vi "LabVIEW host computer v1.0.vi"() -> ()   [LabVIEW 2015]
uses:
  <vilib>/Instr/_visa.llb/VISA Configure Serial Port (Instr).vi
panel:
  out "CH1/CH2":dbl
  out "ch2 dBm":dbl(graph)
  out "XW":string
  out "ch2 Power":dbl(graph)
  out "ch2 Power":dbl
  out "ch2 dB":dbl(graph)
  out "ch2 dB":dbl
  out "ch2 dBm":dbl
  in  "baud rate (9600)":u32=9600 caption="波特率"
  out "XW":string
  out "ch1 Power":dbl(graph)
  out "ch1 Power":dbl
  out "ch1 dB":dbl(graph)
  out "ch1 dB":dbl
  out "ch1 dBm":dbl
  out "ch1 dBm":dbl(graph)
  in  "停止":bool
  in  "VISA resource name":refnum<visa-resource-name> caption="VISA资源名称"
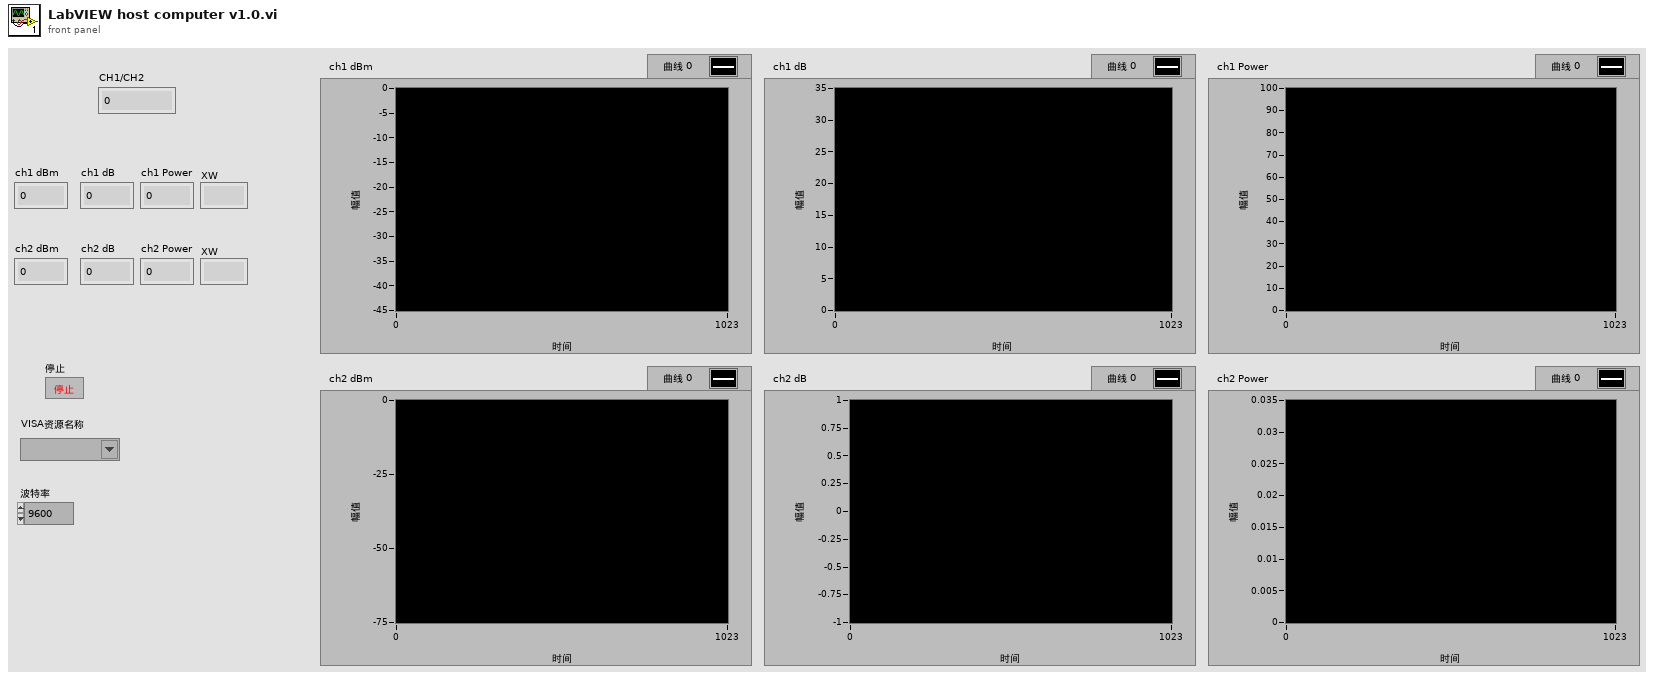
[diagram p1: front panel]
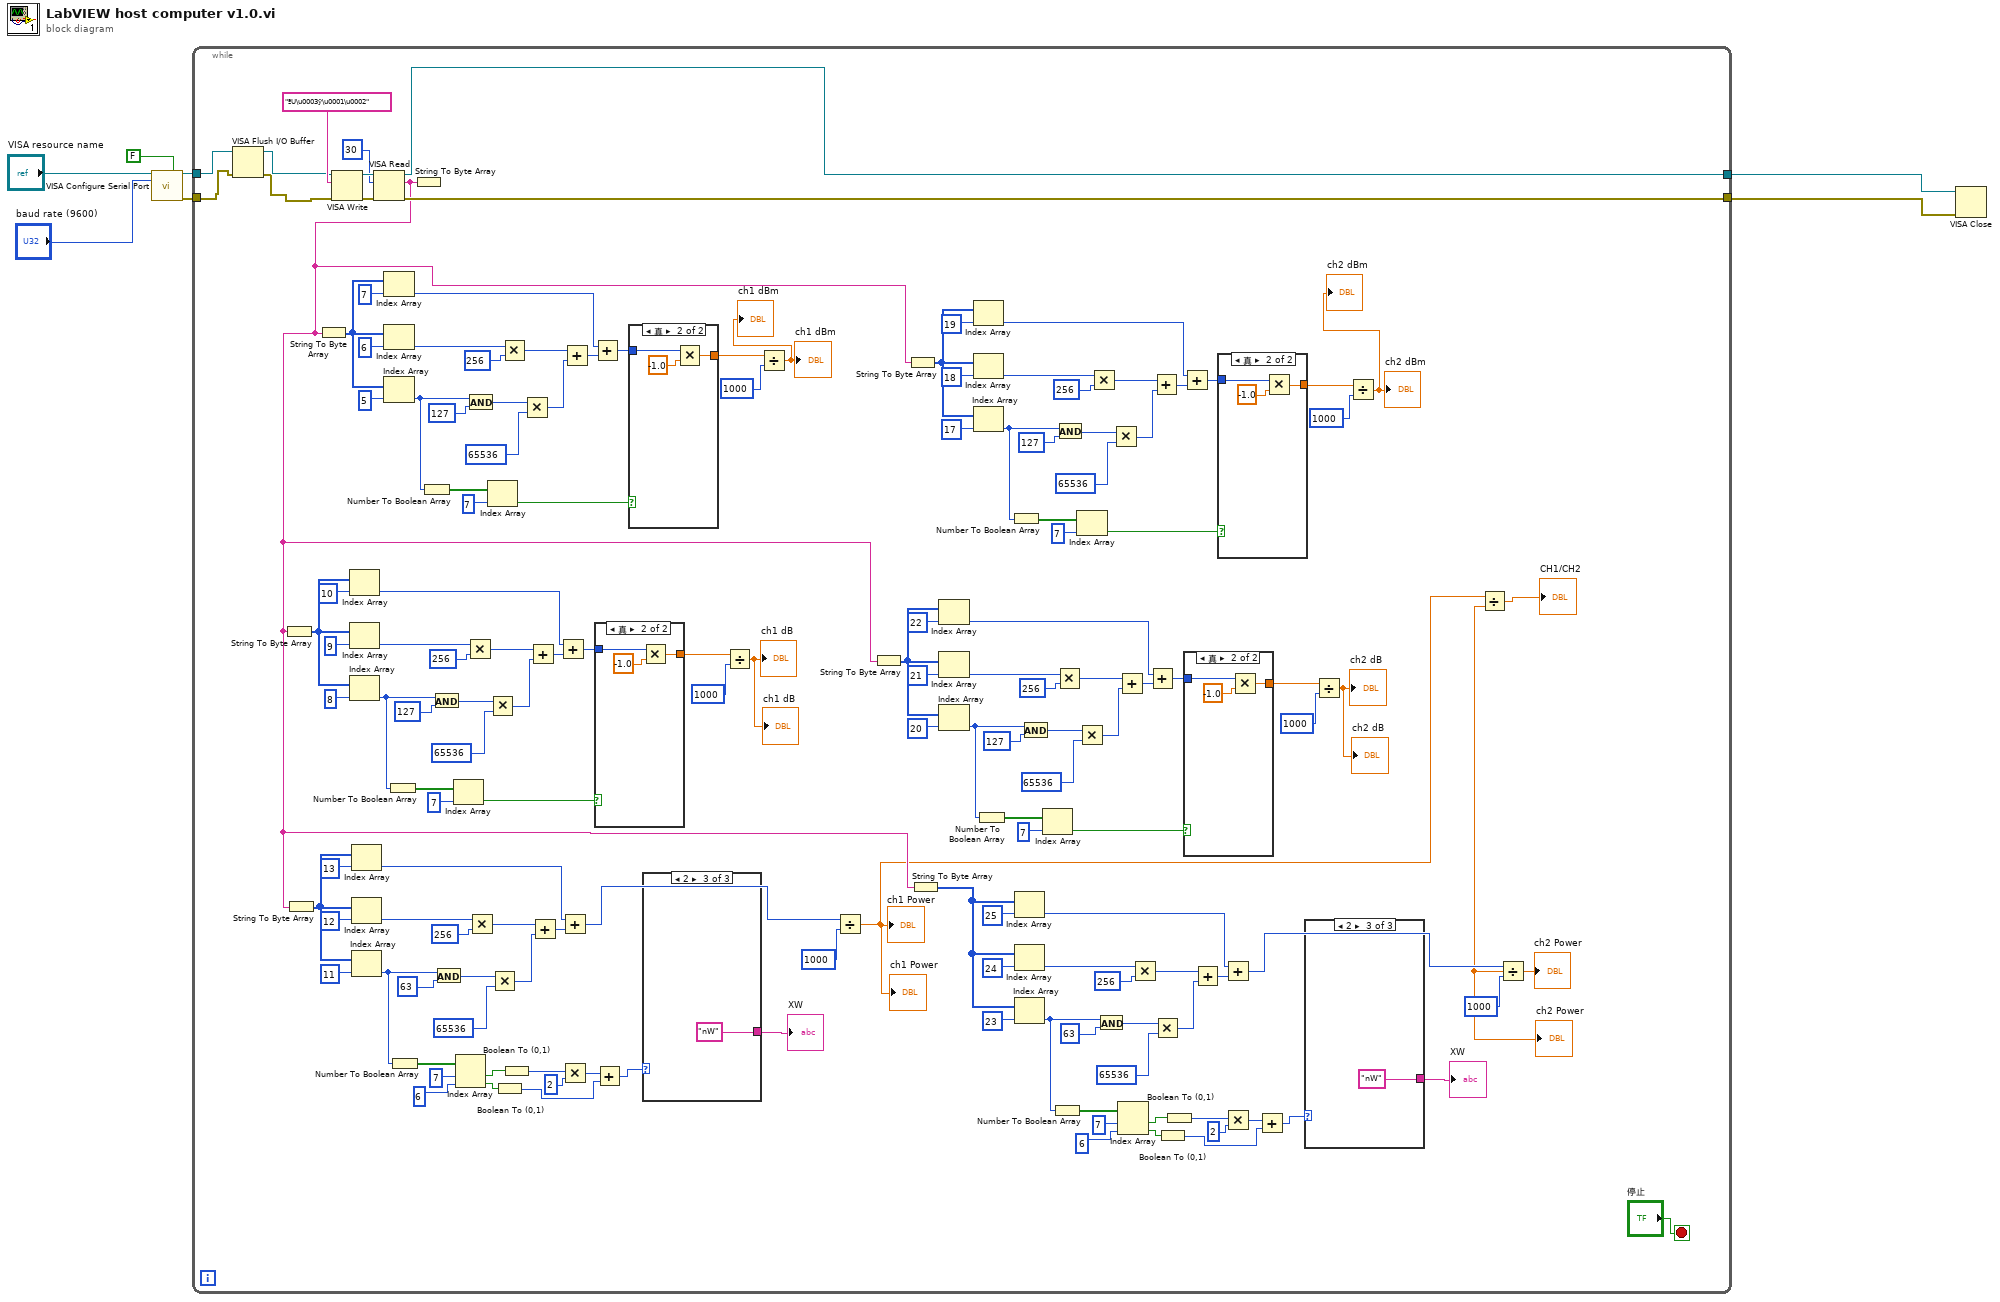
[diagram p0: block diagram]
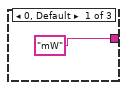
[diagram p2: hidden frame]
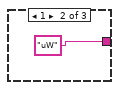
[diagram p3: hidden frame]
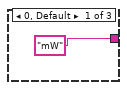
[diagram p6: hidden frame]
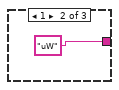
[diagram p7: hidden frame]
diagram:
  n1 = call-poly "VISA Configure Serial Port"("VISA resource name"="VISA resource name", "Enable Termination\nChar (T)"=FALSE ("Enable Termination\nChar (T)"), "baud rate (9600)"="baud rate (9600)") -> ("VISA resource name out"=w5:refnum<visa-resource-name>, "error out"=w4:errorcluster)  [unwired: 11 in]
  n2 = while {
    tunnel: w5 -> [w82]
    tunnel: w4 -> [w85]
    tunnel: [w156] -> w3
    tunnel: [w155] -> w2
    stop <- "停止" stop-if-true
    n3 = VISA Flush I/O Buffer(VISA resource name=w82, error in (no error)=w85) -> (VISA resource name out=w84:refnum<visa-resource-name>, error out=w83:errorcluster)  [unwired: 1 in]
    n4 = VISA Write(VISA resource name=w84, write buffer="ªU\u0003ÿ\u0001\u0002" ("写入缓冲区"), error in (no error)=w83) -> (VISA resource name out=w159:refnum<visa-resource-name>, error out=w158:errorcluster)  [unwired: 1 out]
    n5 = VISA Read(VISA resource name=w159, byte count=u32 30 ("字节总数"), error in (no error)=w158) -> (VISA resource name out=w156:refnum<visa-resource-name>, read buffer=w12:string, error out=w155:errorcluster)  [unwired: 1 out]
    n6 = String To Byte Array(string=w12) -> (unsigned byte array=w132:u8[])
    n7 = String To Byte Array(string=w12) -> (unsigned byte array=w111:u8[])
    n8 = String To Byte Array(string=w12) -> (unsigned byte array=w152:u8[])
    n9 = Index Array(array=w132, index=10) -> (element=w114:u8)
    n10 = Index Array(array=w132, index=9) -> (element=w120:u8)
    n11 = Index Array(array=w132, index=8) -> (element=w126:u8)
    n12 = Index Array(array=w111, index=13) -> (element=w96:u8)
    n13 = Index Array(array=w111, index=12) -> (element=w102:u8)
    n14 = Index Array(array=w111, index=11) -> (element=w108:u8)
    n15 = Index Array(array=w152, index=7) -> (element=w134:u8)
    n16 = Index Array(array=w152, index=6) -> (element=w140:u8)
    n17 = Index Array(array=w152, index=5) -> (element=w146:u8)
    n18 = Number To Boolean Array(number=w126) -> (Boolean array=w127:bool[])
    n19 = Number To Boolean Array(number=w108) -> (Boolean array=w109:bool[])
    n20 = String To Byte Array(string=w12) -> ()  [unwired: 1 out]
    n21 = Number To Boolean Array(number=w146) -> (Boolean array=w147:bool[])
    n22 = And(x=w126, y=127) -> (x .and. y?=w118:i32)
    n23 = And(x=w108, y=63) -> (x .and. y?=w100:i32)
    n24 = Index Array(array=w127, index=7) -> (element=w129:bool)
    n25 = Index Array(array=w109, index #1=7 ("index"), index #2=6 ("索引")) -> (element #1=w94:bool, element #2=w92:bool)
    n26 = Multiply(x=w120, y=u32 256) -> (x*y=w122:u32)
    n27 = And(x=w146, y=127) -> (x .and. y?=w138:i32)
    n28 = Multiply(x=w102, y=u32 256) -> (x*y=w104:u32)
    n29 = Index Array(array=w147, index=7) -> (element=w149:bool)
    n30 = Multiply(x=w118, y=u32 65536) -> (x*y=w123:u32)
    n31 = Multiply(x=w100, y=u32 65536) -> (x*y=w105:u32)
    n32 = Boolean To (0,1)(Boolean=w92) -> (0, 1=w89:i16)
    n33 = Multiply(x=w140, y=u32 256) -> (x*y=w142:u32)
    n34 = Boolean To (0,1)(Boolean=w94) -> (0, 1=w93:i16)
    n35 = Multiply(x=w138, y=u32 65536) -> (x*y=w143:u32)
    n36 = Add(x=w122, y=w123) -> (x+y=w124:u32)
    n37 = Add(x=w104, y=w105) -> (x+y=w106:u32)
    n38 = Add(x=w114, y=w124) -> (x+y=w130:u32)
    n39 = Add(x=w96, y=w106) -> (x+y=w87:u32)
    n40 = Multiply(x=w93, y=2 ("index")) -> (x*y=w90:i32)
    n41 = Add(x=w142, y=w143) -> (x+y=w144:u32)
    n42 = Add(x=w134, y=w144) -> (x+y=w150:u32)
    n43 = case shown="真" w129 {
      tunnel: w130 -> [w175 w178]
      tunnel: [w175 w176] -> w131
      frame False {
      }
      frame True {
        n44 = Multiply(x=w178, y=-1.0) -> (x*y=w176:dbl)
      }
    }
    n45 = Add(x=w90, y=w89) -> (x+y=w88:i32)
    n46 = case shown="真" w149 {
      tunnel: w150 -> [w179 w182]
      tunnel: [w179 w180] -> w151
      frame False {
      }
      frame True {
        n47 = Multiply(x=w182, y=-1.0) -> (x*y=w180:dbl)
      }
    }
    n48 = case shown="2" w88 {
      tunnel: ["mW" "uW" "nW"] -> w86
      frame 0, Default {
      }
      frame 1 {
      }
      frame 2 {
      }
    }
    "XW" <- w86
    n49 = Divide(x=w131, y=u32 1000) -> (x/y=→"ch1 dB" →"ch1 dB":dbl)
    n50 = Divide(x=w151, y=u32 1000) -> (x/y=→"ch1 dBm" →"ch1 dBm":dbl)
    n51 = Divide(x=w87, y=u32 1000) -> (x/y=w9:dbl)
    "ch1 Power" <- w9
    "ch1 Power" <- w9
    n52 = String To Byte Array(string=w12) -> (unsigned byte array=w60:u8[])
    n53 = String To Byte Array(string=w12) -> (unsigned byte array=w80:u8[])
    n54 = String To Byte Array(string=w12) -> (unsigned byte array=w39:u8[])
    n55 = Index Array(array=w60, index=22) -> (element=w42:u8)
    n56 = Index Array(array=w60, index=21) -> (element=w48:u8)
    n57 = Index Array(array=w60, index=20) -> (element=w54:u8)
    n58 = Index Array(array=w80, index=19) -> (element=w62:u8)
    n59 = Index Array(array=w80, index=18) -> (element=w68:u8)
    n60 = Index Array(array=w80, index=17) -> (element=w74:u8)
    n61 = Number To Boolean Array(number=w54) -> (Boolean array=w55:bool[])
    n62 = Number To Boolean Array(number=w74) -> (Boolean array=w75:bool[])
    n63 = Index Array(array=w39, index=25) -> (element=w24:u8)
    n64 = Index Array(array=w39, index=24) -> (element=w30:u8)
    n65 = Index Array(array=w39, index=23) -> (element=w36:u8)
    n66 = And(x=w54, y=127) -> (x .and. y?=w46:i32)
    n67 = Index Array(array=w55, index=7) -> (element=w57:bool)
    n68 = Number To Boolean Array(number=w36) -> (Boolean array=w37:bool[])
    n69 = Multiply(x=w48, y=u32 256) -> (x*y=w50:u32)
    n70 = And(x=w74, y=127) -> (x .and. y?=w66:i32)
    n71 = Index Array(array=w75, index=7) -> (element=w77:bool)
    n72 = Multiply(x=w46, y=u32 65536) -> (x*y=w51:u32)
    n73 = Multiply(x=w68, y=u32 256) -> (x*y=w70:u32)
    n74 = And(x=w36, y=63) -> (x .and. y?=w28:i32)
    n75 = Multiply(x=w66, y=u32 65536) -> (x*y=w71:u32)
    n76 = Add(x=w50, y=w51) -> (x+y=w52:u32)
    n77 = Index Array(array=w37, index #1=7 ("index"), index #2=6 ("索引")) -> (element #1=w22:bool, element #2=w20:bool)
    n78 = Multiply(x=w30, y=u32 256) -> (x*y=w32:u32)
    n79 = Add(x=w42, y=w52) -> (x+y=w58:u32)
    n80 = Add(x=w70, y=w71) -> (x+y=w72:u32)
    n81 = Multiply(x=w28, y=u32 65536) -> (x*y=w33:u32)
    n82 = Boolean To (0,1)(Boolean=w20) -> (0, 1=w17:i16)
    n83 = Boolean To (0,1)(Boolean=w22) -> (0, 1=w21:i16)
    n84 = Add(x=w62, y=w72) -> (x+y=w78:u32)
    n85 = case shown="真" w57 {
      tunnel: w58 -> [w164 w167]
      tunnel: [w164 w165] -> w59
      frame False {
      }
      frame True {
        n86 = Multiply(x=w167, y=-1.0) -> (x*y=w165:dbl)
      }
    }
    n87 = Add(x=w32, y=w33) -> (x+y=w34:u32)
    n88 = case shown="真" w77 {
      tunnel: w78 -> [w168 w171]
      tunnel: [w168 w169] -> w79
      frame False {
      }
      frame True {
        n89 = Multiply(x=w171, y=-1.0) -> (x*y=w169:dbl)
      }
    }
    n90 = Add(x=w24, y=w34) -> (x+y=w15:u32)
    n91 = Multiply(x=w21, y=2 ("index")) -> (x*y=w18:i32)
    n92 = Add(x=w18, y=w17) -> (x+y=w16:i32)
    n93 = case shown="2" w16 {
      tunnel: ["mW" "uW" "nW"] -> w14
      frame 0, Default {
      }
      frame 1 {
      }
      frame 2 {
      }
    }
    "XW" <- w14
    n94 = Divide(x=w59, y=u32 1000) -> (x/y=→"ch2 dB" →"ch2 dB":dbl)
    n95 = Divide(x=w79, y=u32 1000) -> (x/y=→"ch2 dBm" →"ch2 dBm":dbl)
    n96 = Divide(x=w15, y=u32 1000) -> (x/y=w8:dbl)
    "ch2 Power" <- w8
    "ch2 Power" <- w8
    n97 = Divide(x=w9, y=w8) -> (x/y=→"CH1/CH2":dbl)
  }
  n98 = VISA Close(VISA resource name=w3, error in (no error)=w2) -> ()  [unwired: 1 out]
